vi "cross_correlate.vi"(4 "Ref Image Cropped":T1, 5 "Template Image Cropped":T1, 6 "Template Height":i32=50, 7 "Depth":i32=50, 8 "Template Width":i32=200, 9 "Vertical Search Range":i32=50, 10 "Ref Image":T1, 11 "Template Image":T1) -> (0 "template coordinates":i32[](array[numeric]), 1 "score":dbl, 2 "y shift":i32, 3 "x shift":i32)   [LabVIEW 2016]
doc: "Registers two images using normalised cross correlation. Extracts template from image and calculates norm x corr with reference image. X Shift and Y Shift and correlation value are reported. Using Fast Match which uses the OpenCV norm x corr function."
uses:
  <vilib>/vision/Image Controls.llb/IMAQ Image.ctl
panel:
  out "Top Limit":i32=50
  out "Bottom Limi":i32
  out "Chosen":i32
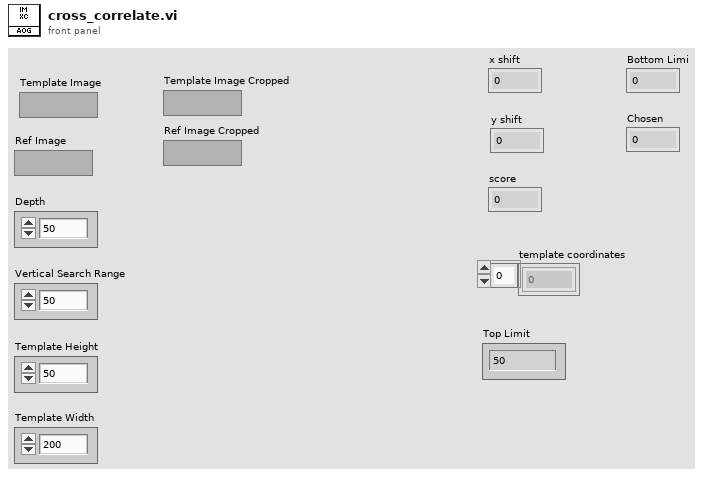
[diagram p1: front panel]
types:
  T1 = typedef "IMAQ Image.ctl" = refnum<image>
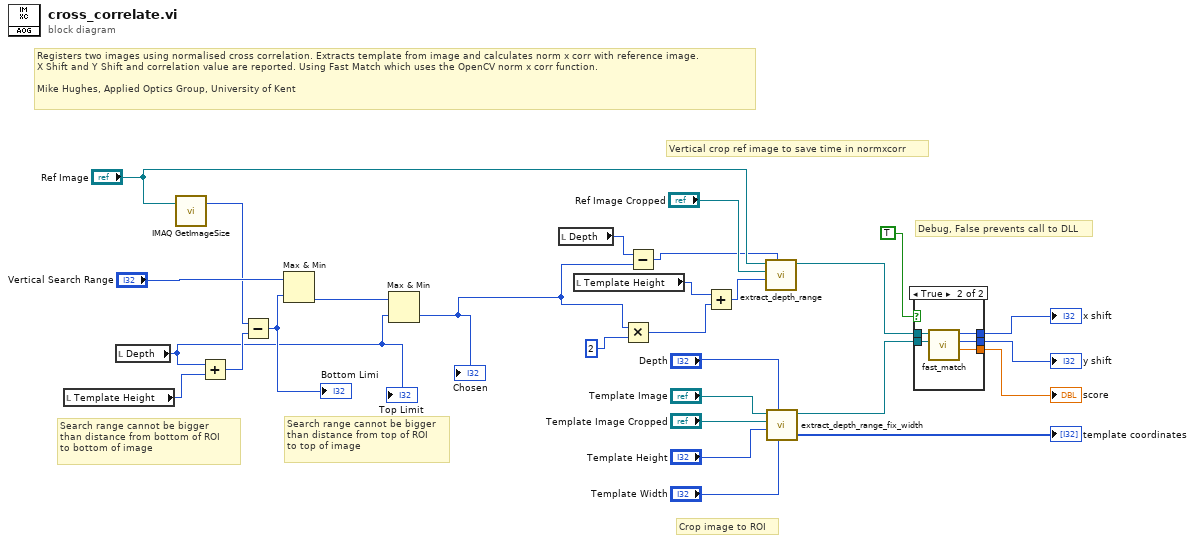
[diagram p0: block diagram]
diagram:
  # "Search range cannot be bigger\nthan distance from top of ROI\nto top of image"
  # "Search range cannot be bigger\nthan distance from bottom of ROI\nto bottom of image"
  # "Crop image to ROI"
  # "Vertical crop ref image to save time in normxcorr"
  # "Debug, False prevents call to DLL"
  # "Registers two images using normalised cross correlation. Extracts template from image and calculates norm x corr with reference image.\nX Shift and Y Shift and correlation value are reported. Using Fast Match which uses the OpenCV norm x corr function.\n\nMike Hughes, Applied Optics Group, University of Kent"
  n1 = local read "Template Height"() -> (w12:i32)
  n2 = local read "Depth"() -> (w8:i32)
  "Top Limit" <- w8
  n3 = call "IMAQ GetImageSize"("Image"="Ref Image") -> ("Y Resolution"=w11:i32)  [unwired: 3 in, 2 out]
  n4 = Add(x=w8, y=w12) -> (x+y=w10:i32)
  n5 = Subtract(x=w11, y=w10) -> (x-y=w9:i32)
  "Bottom Limi" <- w9
  n6 = Max & Min(x="Vertical Search Range", y=w9) -> (min(x,y)=w13:i32)  [unwired: 1 out]
  n7 = Max & Min(x=w13, y=w8) -> (min(x,y)=w2:i32)  [unwired: 1 out]
  "Chosen" <- w2
  n8 = local read "Depth"() -> (w6:i32)
  n9 = local read "Template Height"() -> (w1:i32)
  n10 = Multiply(x=w2, y=2 ("x")) -> (x*y=w3:i32)
  n11 = Subtract(x=w6, y=w2) -> (x-y=w5:i32)
  n12 = Add(x=w1, y=w3) -> (x+y=w7:i32)
  n13 = call "extract_depth_range.vi"("offset"=w5, "size"=w7, "Image Dst"="Ref Image Cropped", "Image"="Ref Image") -> ("Image Dst Out"=w24:T1)  [unwired: 6 in, 1 out]
  n14 = call "extract_depth_range_fix_width.vi"("width"="Template Width", "vertical offset"="Depth", "vertical size"="Template Height", "Image Dst"="Template Image Cropped", "Image"="Template Image") -> ("co-ordinates"=→"template coordinates":i32[], "Image Dst Out"=w23:T1)  [unwired: 4 in, 1 out]
  n15 = case shown="True" TRUE {
    tunnel: w24 -> [_ w33]
    tunnel: w23 -> [_ w32]
    tunnel: [_ w31] -> w22
    tunnel: [_ w30] -> w21
    tunnel: [_ w29] -> w20
    frame False {
    }
    frame True {
      n16 = call "fast_match.vi"("Template"=w32, "Image"=w33) -> ("score"=w29:dbl, "y shift"=w30:i32, "x shift"=w31:i32)  [unwired: 6 in, 1 out]
    }
  }
  "x shift" <- w22
  "y shift" <- w21
  "score" <- w20
